vi "Constant - CSV Header.vi"() -> (2 "CSV Header":string)   [LabVIEW 2021]
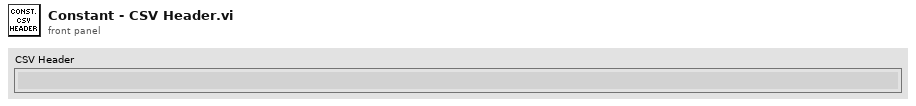
[diagram p1: front panel]
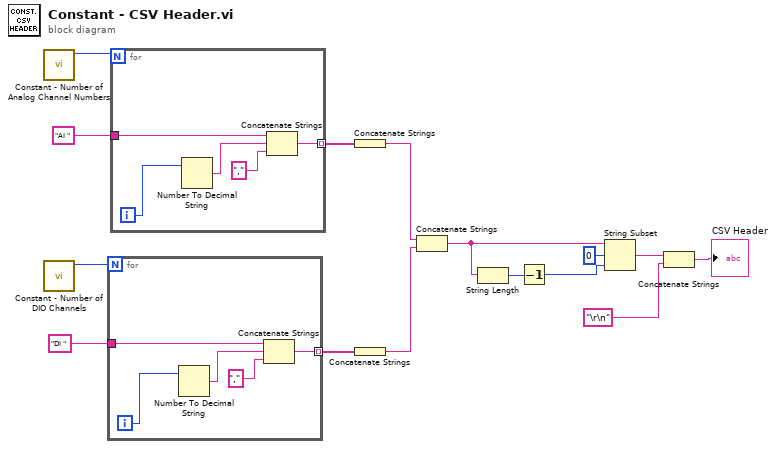
[diagram p0: block diagram]
diagram:
  n1 = call "Constant - Number of Analog Channel Numbers.vi"() -> ("Maximum Channel"=w14:i32)  [unwired: 11 in]
  n2 = call "Constant - Number of DIO Channels.vi"() -> ("Maximum Channel"=w11:i32)  [unwired: 11 in]
  n3 = for {
    N: w11 -> [_]
    tunnel: "DI " -> [w20]
    tunnel: [w16] -> w10 mode=indexing
    i -> [w19]
    n4 = Number To Decimal String(number=w19) -> (decimal integer string=w18:string)  [unwired: 1 in]
    n5 = Concatenate Strings(w20, w18, "," ("string")) -> (w16:string)
  }
  n6 = for {
    N: w14 -> [_]
    tunnel: "AI " -> [w25]
    tunnel: [w21] -> w13 mode=indexing
    i -> [w24]
    n7 = Number To Decimal String(number=w24) -> (decimal integer string=w23:string)  [unwired: 1 in]
    n8 = Concatenate Strings(w25, w23, "," ("string")) -> (w21:string)
  }
  n9 = Concatenate Strings(w13) -> (w9:string)
  n10 = Concatenate Strings(w10) -> (w8:string)
  n11 = Concatenate Strings(w9, w8) -> (w7:string)
  n12 = String Length(string=w7) -> (length=w6:i32)
  n13 = Decrement(x=w6) -> (x-1=w5:i32)
  n14 = String Subset(string=w7, offset (0)=0, length (rest)=w5) -> (substring=w2:string)
  n15 = Concatenate Strings(w2, "\r\n" ("string")) -> (→"CSV Header":string)
